vi "Tokenizer.vi"(0 "Tokenizer sequence":string, 2 "Input string":string) -> (16 "Text segments":string[](array[string]))   [LabVIEW 2026]
doc: "This VI returns single lines from input string. If number of lines (Array size) is known, algorithm is faster, otherwise Array size = 0 should be used. Sub-VI for VST?.vi and Define macro contents (with or without) delay.vi."
uses:
  <vilib>/regexp/Match Regular Expression.xnode
panel:
  # "String tokenizer to split text segments with given tokenizer sequence."
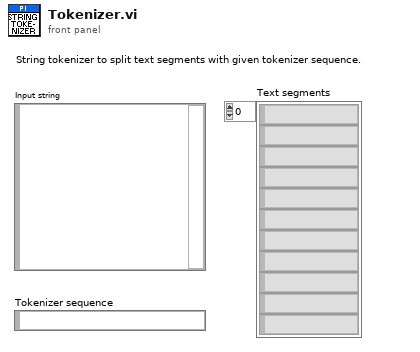
[diagram p1: front panel]
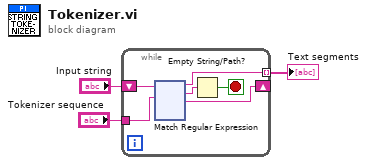
[diagram p0: block diagram]
diagram:
  n1 = while {
    shift-right: [w9] -> _
    shift-left: "Input string" -> [w5]
    tunnel: [w8] -> w2 mode=indexing
    tunnel: "Tokenizer sequence" -> [w4]
    stop <- w6 stop-if-true
    n2 = xnode "Match Regular Expression"("chaîne en entrée"=w5, "expression régulière"=w4) -> ("avant la correspondance"=w8:string, "toute l'expression"=w7:string, "après la correspondance"=w9:string)  [unwired: 4 in, 2 out]
    n3 = Empty String/Path?(string/path=w7) -> (empty?=w6:bool)
  }
  "Text segments" <- w2
